vi "Create_Raw_data_file.vi"(4 "No of averages":i32=1, 5 "End time":dbl, 6 "Start time":dbl, 7 "Setup filename":string) -> (0 "Error String":string, 1 "Values":string[][](array[string]), 2 "Header Comments":string[](array[string]), 3 "Column headers":string[](array[string]))   [LabVIEW 2014]
uses:
  File/Setup_Filetype.ctl
  Controls/Post_Process.ctl
  Globals/Preference_global.vi
  Globals/Meas_global.vi
  Globals/Trav_pos_global.vi
  Globals/Constants_global.vi
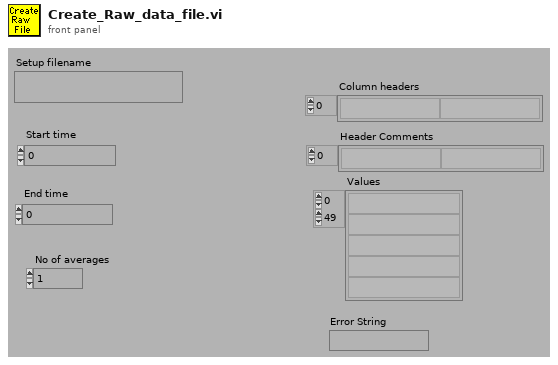
[diagram p1: front panel]
types:
  T1 = typedef "Post_Process.ctl" = enum16{"Take New Data", "Post Process Raw Data File"}
  T2 = typedef "Server_Comms.ctl" = enum16{"Server Link Healthy", "Do Not Link To Server"}
  T3 = typedef "Setup_Filetype.ctl" = enum16{"Measurement Setups", "Calibration Setups", "General", "Results File Plotter Setups", "Speed Calib Tweaks"}
  T4 = typedef "Traverse_cluster.ctl" = cluster{"Start X":sgl, "Start Y":sgl, "Start Z":sgl, "End X":sgl, "End Y":sgl, "End Z":sgl, "No. of pts.":i32, "Spacing":T5, "Filename":path, "Tunnel Speed":dbl, "Averaging time (min)":dbl, "Extra Commands":string, "Carrier_1 Q (l/min)":dbl, "Carrier_2 Q (l/min)":dbl, "Trace Gas Concentration (%)":dbl, "Specific Arguments":string, "Comments":string, "Row No":i32, "Row Type Selector":T6, "Completion time":string, "Row Duration (mins)":dbl, "No. of Valid pts.":i32, "Meas Setup File":string}
  T5 = typedef "Spacing.ctl" = enum16{"Linear", "Log", "Gauss", "Specified", "N/A"}
  T6 = typedef "Multi_run_mode.ctl" = enum16{"Move Traverse Only", "Set Tunnel Speed Only", "Set Source Only", "Set Measurement Conditions", "Single Measurement", "Vertical Profile", "Lateral Profile", "Longitudinal Profile", "Explore Volume", "Multi-Axis Profile", "Auto Calibrate", "Meas Fast FID Bkgnd", "Check Beam Power", "Scanning Valve Measurement", "Run VI Named:", "Set ADAM Ch", "Wait (minutes)", "Send Message", "Synchronize With:", "Fall Back to this Row", "Turn Off Row Repeating", "Blank Row", "Traverse 3D Volume"}
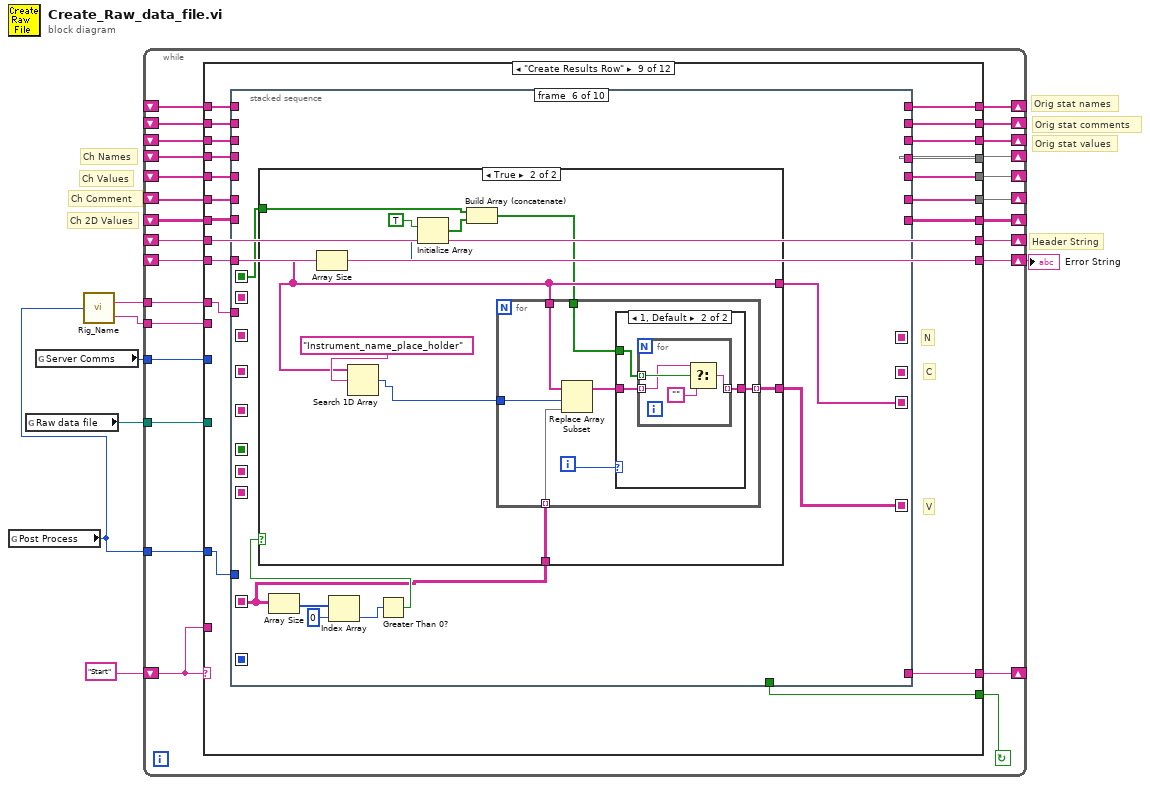
[diagram p0: block diagram]
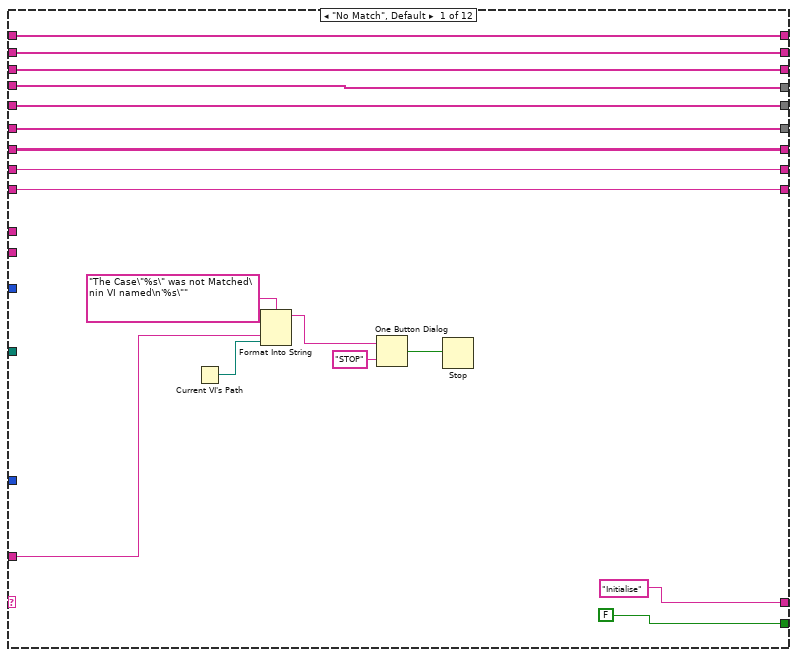
[diagram p2: hidden frame]
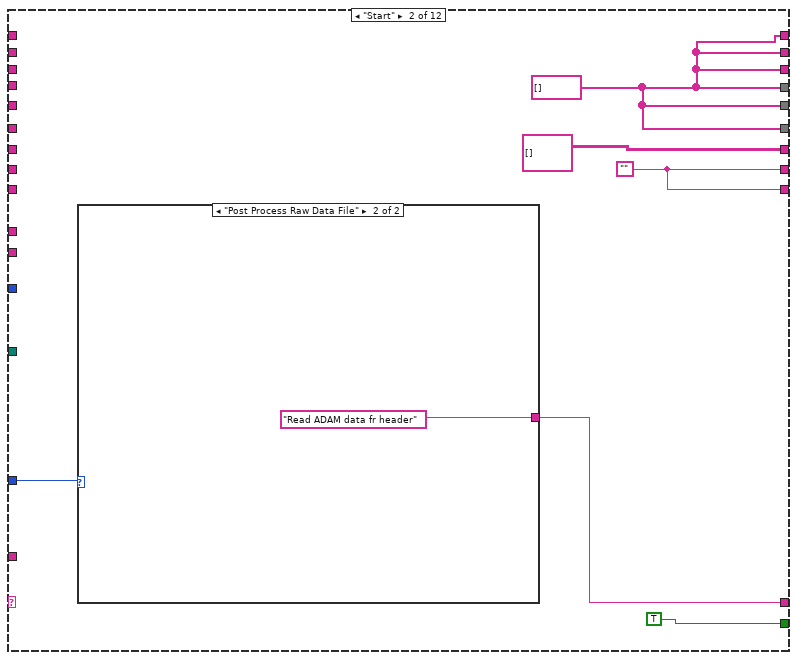
[diagram p3: hidden frame]
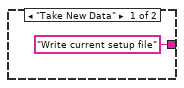
[diagram p4: hidden frame]
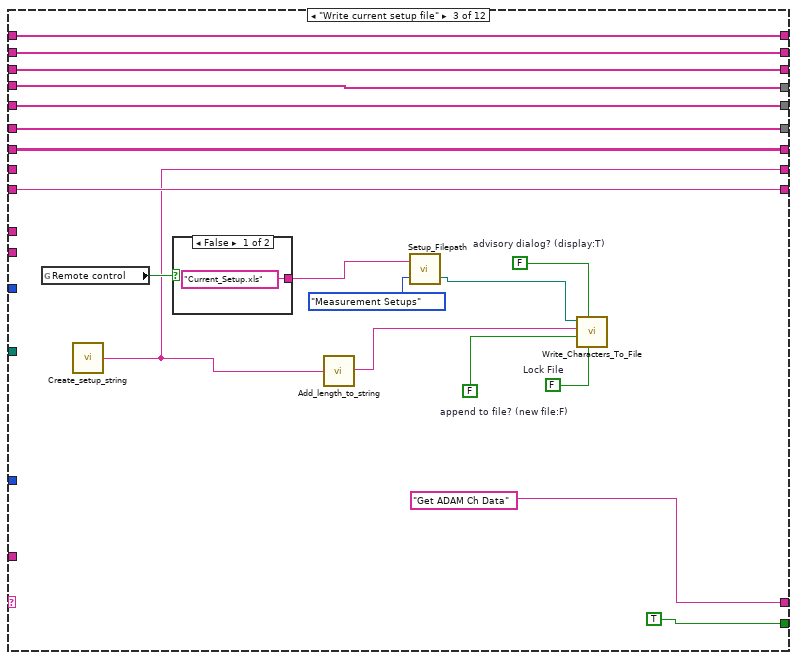
[diagram p5: hidden frame]
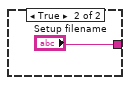
[diagram p6: hidden frame]
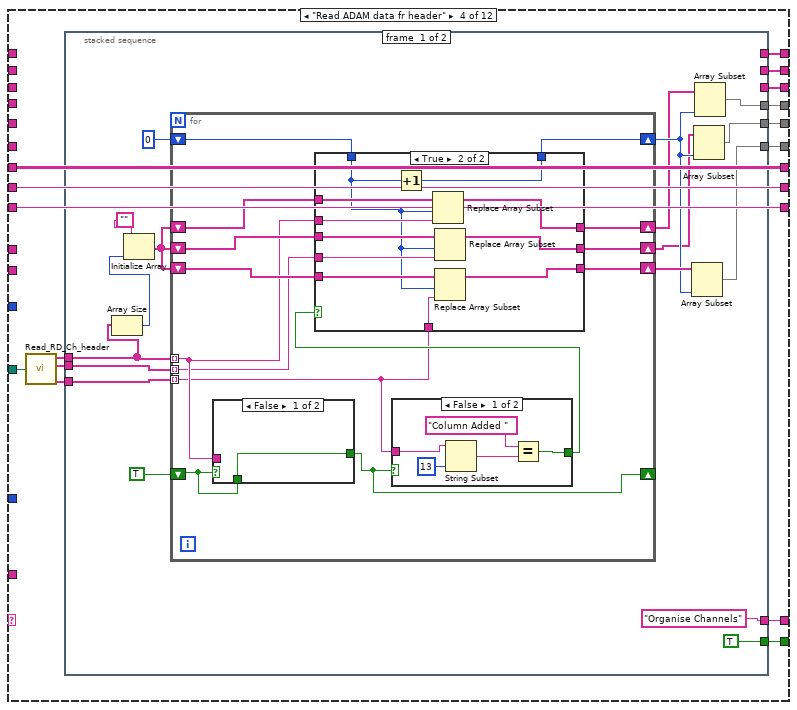
[diagram p7: hidden frame]
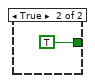
[diagram p9: hidden frame]
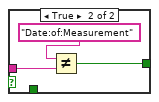
[diagram p10: hidden frame]
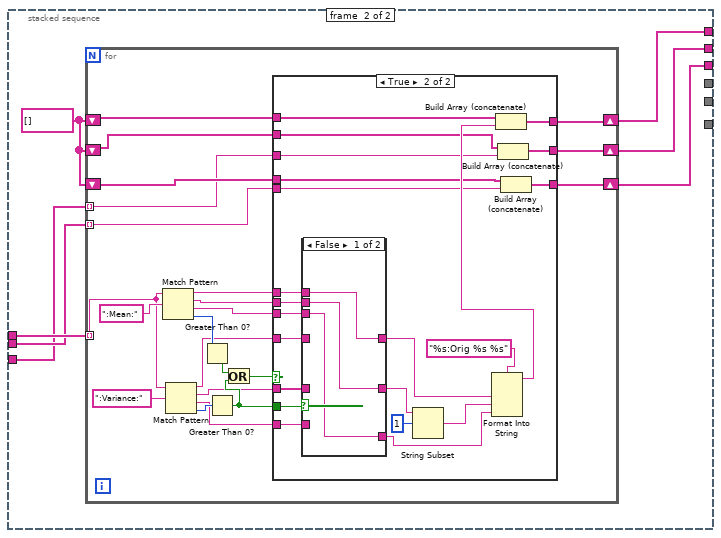
[diagram p11: hidden frame]
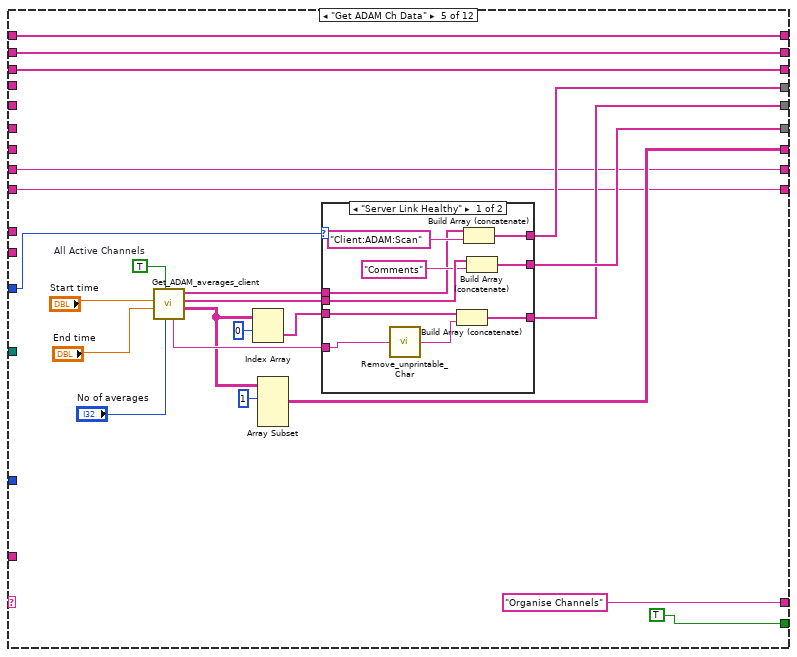
[diagram p14: hidden frame]
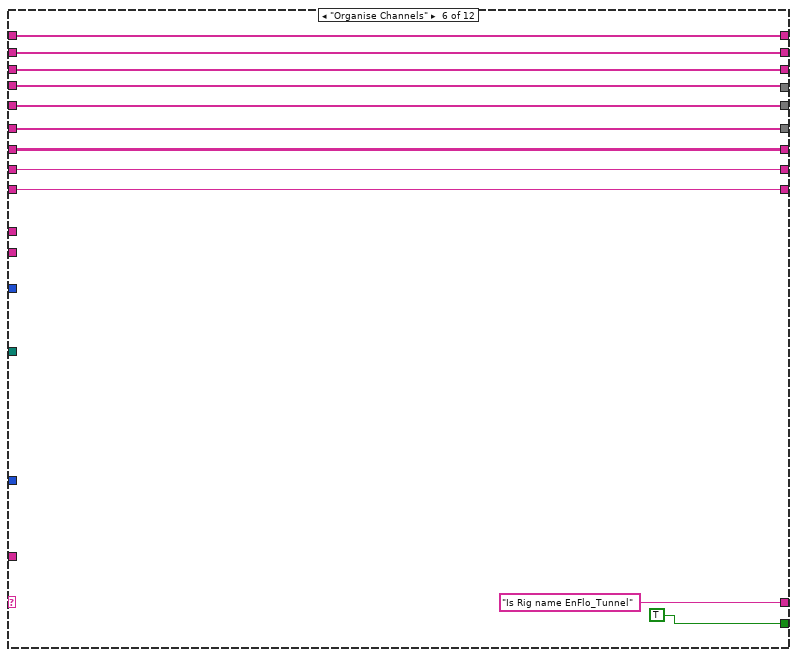
[diagram p16: hidden frame]
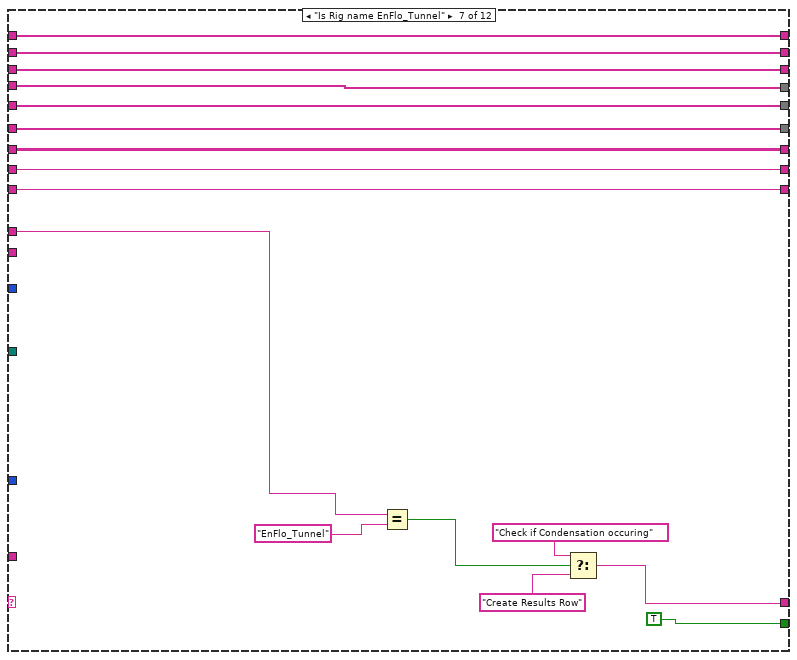
[diagram p17: hidden frame]
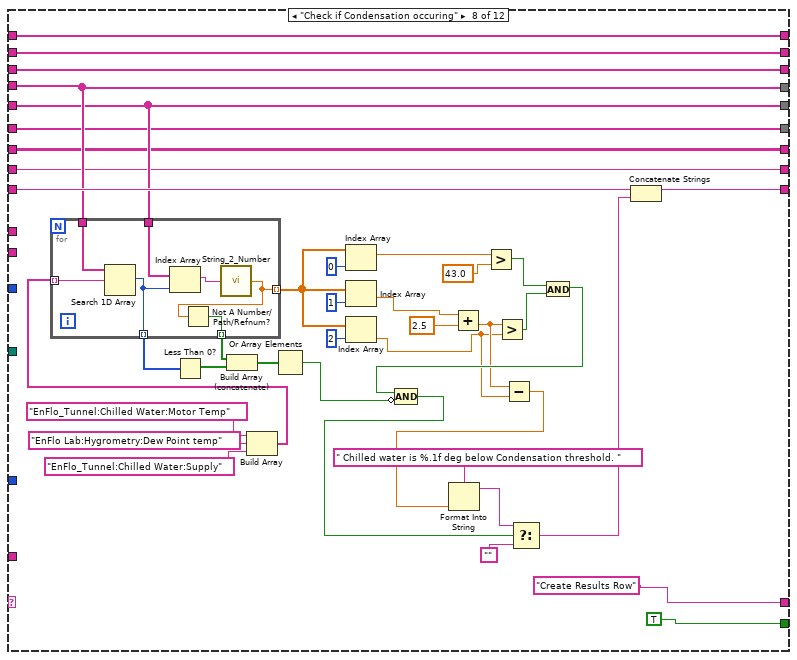
[diagram p18: hidden frame]
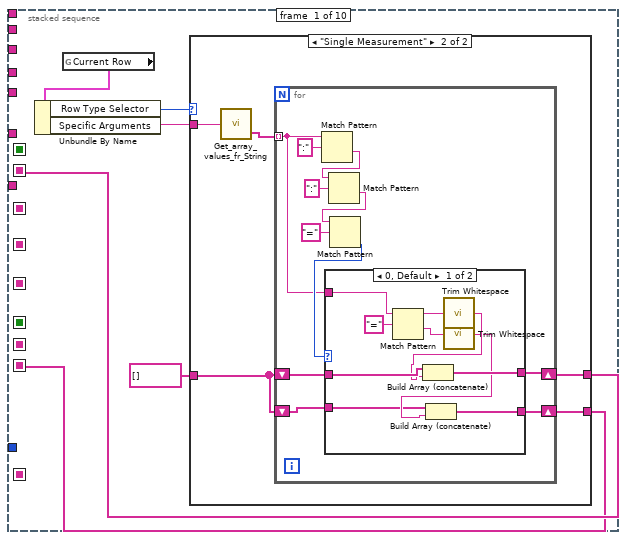
[diagram p19: hidden frame]
diagram:
  # "Orig stat values"
  # "Orig stat comments"
  # "Orig stat names"
  # "Header String"
  # "Ch 2D Values"
  # "Ch Comment"
  # "Ch Values"
  # "Ch Names"
  n1 = global read "Meas_global.vi" "Post Process"() -> (w3:T1)
  n2 = global read "Meas_global.vi" "Raw data file"() -> (w6:path)
  n3 = global read "Preference_global.vi" "Server Comms"() -> (w5:T2)
  n4 = call "Rig_Name.vi"("Post Process"=w3) -> ("Rig Setup before dash"=w2:string, "Hard Disk name"=w1:string)
  n5 = while {
    tunnel: w5 -> [w16]
    tunnel: w6 -> [w17]
    tunnel: w3 -> [w18]
    shift-left: _ -> [w20]
    shift-right: [w19] -> _
    shift-left: _ -> [w26]
    shift-right: [w25] -> w4
    shift-left: _ -> [w21]
    shift-right: [w27] -> _
    shift-left: _ -> [w22]
    shift-right: [w29] -> _
    shift-left: _ -> [w23]
    shift-right: [w28] -> _
    shift-left: _ -> [w24]
    shift-right: [w30] -> _
    shift-left: "Start" -> [w31]
    shift-right: [w32] -> _
    tunnel: w2 -> [w15]
    tunnel: w1 -> [w14]
    shift-right: [w10] -> _
    shift-left: _ -> [w11]
    shift-right: [w8] -> _
    shift-left: _ -> [w9]
    shift-right: [w12] -> _
    shift-left: _ -> [w13]
    stop <- w33 continue-if-true
    n6 = case shown="\"Create Results Row\"" w31 {
      tunnel: [FALSE TRUE TRUE w83 TRUE TRUE TRUE TRUE w328 TRUE TRUE FALSE] -> w33
      tunnel: ["Initialise" w52 "Get ADAM Ch Data" w94 "Organise Channels" "Is Rig name EnFlo_Tunnel" w265 "Create Results Row" w340 "Add Raw Data header info" "Add Raw Data fr Tempory file" "End"] -> w32
      tunnel: w31 -> [w45 _ _ _ _ _ _ _ _ _ _ _]
      tunnel: [w42 w51 w77 w85 w221 w255 w273 w283 w337 w643 w673 w690] -> w30
      tunnel: [w40 w51 w75 w86 w220 w253 w271 w281 w334 w654 w675 w692] -> w29
      tunnel: [w41 w51 w76 w84 w219 w254 w272 w282 w330 w655 w674 w691] -> w28
      tunnel: [w39 string[][] [] w74 w92 w217 w252 w270 w280 w332 w646 w676 w693] -> w27
      tunnel: w26 -> [w38 _ w72 w93 w216 w250 w267 w286 w338 w659 w677 w694]
      tunnel: [w38 w54 w72 w93 w216 w250 w267 w284 w338 w659 w677 w694] -> w25
      tunnel: w24 -> [w42 _ w77 _ _ w255 w273 w283 w336 w643 w673 w690]
      tunnel: w23 -> [w41 _ w76 _ _ w254 w272 w282 w331 w655 w674 w691]
      tunnel: w22 -> [w40 _ w75 _ _ w253 w271 w281 w335 w654 w675 w692]
      tunnel: w21 -> [w39 _ w74 w92 _ w252 w270 w280 w333 w646 w676 w693]
      tunnel: w20 -> [w37 _ _ w91 w215 w251 w268 w278 w339 w648 w670 w689]
      tunnel: [w37 w54 w66 w91 w215 w251 w268 w278 w339 w651 w669 ""] -> w19
      tunnel: w18 -> [_ w53 _ _ _ _ _ _ w329 _ _ _]
      tunnel: w17 -> [_ _ _ w90 _ _ _ _ _ _ _ w685]
      tunnel: w16 -> [_ _ _ _ w214 _ _ _ _ _ _ _]
      tunnel: w15 -> [_ _ _ _ _ _ w262 _ w327 _ _ _]
      tunnel: w14 -> [_ _ _ _ _ _ _ _ _ _ _ _]
      tunnel: w13 -> [w36 _ w64 _ w213 w249 w260 w277 w325 w640 w668 w682]
      tunnel: [w36 w51 w64 w82 w213 w249 w260 w277 w326 w640 w668 w682] -> w12
      tunnel: w11 -> [w35 _ w63 _ w212 w248 w259 w276 w324 w639 w667 w681]
      tunnel: [w35 w51 w63 w81 w212 w248 w259 w276 w323 w639 w667 w681] -> w10
      tunnel: w9 -> [w34 _ w62 _ w211 w247 w258 w275 w321 w638 w666 w680]
      tunnel: [w34 w51 w62 w80 w211 w247 w258 w275 w322 w638 w666 w680] -> w8
      frame "No Match", Default {
        n7 = Current VI's Path() -> (path=w44:path)
        n8 = Format Into String(format string="The Case\"%s\" was not Matched\nin VI named\n'%s\"" ("Format String"), w45, w44) -> (resulting string=w48:string)  [unwired: 2 in, 1 out]
        n9 = One Button Dialog(message=w48, button name ("OK")="STOP") -> (true=w46:bool)
        n10 = Stop(stop? (T)=w46) -> ()
      }
      frame "Start" {
        w54 = ""
        w51 = string[] []
        n11 = case shown="\"Post Process Raw Data File\"" w53 {
          tunnel: ["Write current setup file" "Read ADAM data fr header"] -> w52
          frame "Take New Data" {
          }
          frame "Post Process Raw Data File" {
          }
        }
      }
      frame "Write current setup file" {
        w67 = FALSE  # Lock File
        w70 = FALSE  # advisory dialog? (display:T)
        w71 = FALSE  # append to file? (new file:F)
        n12 = global read "Meas_global.vi" "Remote control"() -> (w69:bool)
        n13 = call "Create_setup_string.vi"() -> ("Setup String"=w66:string)  [unwired: 1 out]
        n14 = case shown="False" w69 {
          tunnel: ["Current_Setup.xls" ("Setup filename") "Setup filename"] -> w60
          frame False {
          }
          frame True {
          }
        }
        n15 = call "Add_length_to_string.vi"("String in"=w66) -> ("String out"=w68:string)
        n16 = call "Setup_Filepath.vi"("Setup File Type"=Setup_Filetype."Measurement Setups", "Filename in"=w60) -> ("Filename Out"=w59:path)  [unwired: 1 out]
        n17 = call "Write_Characters_To_File.vi"("file path (dialog if empty)"=w59, "advisory dialog? (display:T)"=w70, "character string"=w68, "append to file? (new file:F)"=w71, "Lock File"=w67) -> ()  [unwired: 4 out]
      }
      frame "Read ADAM data fr header" {
        n18 = call "Read_RD_Ch_header.vi"("Raw data file"=w90) -> ("Ch Name Out"=w88:string[], "Ch Values"=w87:string[], "Comments"=w89:string[])  [unwired: 1 out]
        n19 = stacked-sequence {
          tunnel: ["Organise Channels" _] -> w94
          tunnel: w89 -> [w109 w154]
          tunnel: w88 -> [w108 w157]
          tunnel: w87 -> [w103 w155]
          tunnel: [w100 _] -> w86
          tunnel: [w97 _] -> w85
          tunnel: [w96 _] -> w84
          tunnel: [TRUE _] -> w83
          tunnel: [_ w153] -> w82
          tunnel: [_ w152] -> w81
          tunnel: [_ w151] -> w80
          frame #0 {
            n20 = Array Size(array=w108) -> (size(s)=w106:i32)
            n21 = Initialize Array("", w106) -> (w105:string[])
            n22 = for {
              shift-right: [w112] -> w101
              shift-left: 0 -> [w122]
              shift-right: [w116] -> w102
              shift-left: w105 -> [w119]
              shift-right: [w117] -> w99
              shift-left: w105 -> [w120]
              shift-right: [w118] -> w98
              shift-left: w105 -> [w121]
              shift-right: [w124] -> _
              shift-left: TRUE -> [w125]
              tunnel: w108 -> [w115] mode=indexing
              tunnel: w109 -> [w113] mode=indexing
              tunnel: w103 -> [w114] mode=indexing
              n23 = case shown="False" w125 {
                tunnel: w115 -> [_ w150]
                tunnel: [w147 w148] -> w124
                tunnel: w125 -> [w147 _]
                frame False {
                }
                frame True {
                  n24 = Not Equal?(x="Date:of:Measurement", y=w150) -> (x != y?=w148:bool)
                }
              }
              n25 = case shown="False" w124 {
                tunnel: w113 -> [w142 _]
                tunnel: [w144 TRUE] -> w123
                frame False {
                  n26 = String Subset(string=w142, length (rest)=13 ("length (rest)")) -> (substring=w141:string)  [unwired: 1 out]
                  n27 = Equal?(x="Column Added ", y=w141) -> (x = y?=w144:bool)
                }
                frame True {
                }
              }
              n28 = case shown="True" w123 {
                tunnel: w122 -> [w126 w131]
                tunnel: w121 -> [w129 w140]
                tunnel: w120 -> [w128 w139]
                tunnel: w119 -> [w127 w138]
                tunnel: [w129 w137] -> w118
                tunnel: [w128 w136] -> w117
                tunnel: [w127 w135] -> w116
                tunnel: w115 -> [_ w134]
                tunnel: w114 -> [_ w133]
                tunnel: w113 -> [_ w132]
                tunnel: [w126 w130] -> w112
                frame False {
                }
                frame True {
                  n29 = Increment(x=w131) -> (x+1=w130:i32)
                  n30 = Replace Array Subset(array=w140, new element=w134, index=w131) -> (w137:string[])
                  n31 = Replace Array Subset(array=w139, new element=w133, index=w131) -> (w136:string[])
                  n32 = Replace Array Subset(array=w138, new element=w132, index=w131) -> (w135:string[])
                }
              }
            }
            n33 = Array Subset(array=w102, length=w101) -> (w100:string[])  [unwired: 1 in]
            n34 = Array Subset(array=w99, length=w101) -> (w96:string[])  [unwired: 1 in]
            n35 = Array Subset(array=w98, length=w101) -> (w97:string[])  [unwired: 1 in]
          }
          frame #1 {
            w156 = string[] []
            n36 = for {
              shift-right: [w165] -> w153
              shift-left: w156 -> [w164]
              shift-right: [w158] -> w152
              shift-left: w156 -> [w159]
              shift-right: [w161] -> w151
              shift-left: w156 -> [w162]
              tunnel: w157 -> [w177] mode=indexing
              tunnel: w155 -> [w163] mode=indexing
              tunnel: w154 -> [w160] mode=indexing
              n37 = Match Pattern(string=w177, regular expression=":Mean:") -> (before substring=w168:string, match substring=w167:string, after substring=w166:string, offset past match=w176:i32)  [unwired: 1 out]
              n38 = Match Pattern(string=w177, regular expression=":Variance:") -> (before substring=w171:string, match substring=w170:string, after substring=w169:string, offset past match=w175:i32)  [unwired: 1 out]
              n39 = Greater Than 0?(x=w176) -> (x > 0?=w174:bool)
              n40 = Greater Than 0?(x=w175) -> (x > 0?=w172:bool)
              n41 = Or(x=w174, y=w172) -> (x .or. y?=w173:bool)
              n42 = case shown="True" w173 {
                tunnel: w172 -> [_ w204]
                tunnel: w171 -> [_ w203]
                tunnel: w170 -> [_ w202]
                tunnel: w169 -> [_ w201]
                tunnel: w168 -> [_ w194]
                tunnel: w167 -> [_ w193]
                tunnel: w166 -> [_ w192]
                tunnel: [w182 w190] -> w165
                tunnel: w164 -> [w182 w189]
                tunnel: w163 -> [_ w188]
                tunnel: w162 -> [w180 w187]
                tunnel: [w180 w186] -> w161
                tunnel: w160 -> [_ w185]
                tunnel: w159 -> [w181 w184]
                tunnel: [w181 w183] -> w158
                frame False {
                }
                frame True {
                  n43 = case shown="False" w204 {
                    tunnel: w203 -> [_ w209]
                    tunnel: w202 -> [_ w210]
                    tunnel: w201 -> [_ w208]
                    tunnel: [w206 w210] -> w199
                    tunnel: [w207 w209] -> w196
                    tunnel: [w205 w208] -> w195
                    tunnel: w194 -> [w207 _]
                    tunnel: w193 -> [w206 _]
                    tunnel: w192 -> [w205 _]
                    frame False {
                    }
                    frame True {
                    }
                  }
                  n44 = String Subset(string=w199, offset (0)=1) -> (substring=w198:string)  [unwired: 1 out]
                  n45 = Format Into String(format string="%s:Orig %s %s", w196, w198, w195) -> (resulting string=w191:string)  [unwired: 2 in, 1 out]
                  n46 = Build Array (concatenate)(w189, w191) -> (w190:string[])
                  n47 = Build Array (concatenate)(w184, w185) -> (w183:string[])
                  n48 = Build Array (concatenate)(w187, w188) -> (w186:string[])
                }
              }
            }
          }
        }
      }
      frame "Get ADAM Ch Data" {
        w224 = TRUE  # All Active Channels
        n49 = call "Get_ADAM_averages_client.vi"("No of averages"="No of averages", "All Active Channels"=w224, "End time"="End time", "Start time"="Start time") -> ("Values"=w227:string[][], "Comments"=w230:string[], "Titles"=w229:string[], "Messages"=w231:string)  [unwired: 1 in, 3 out]
        n50 = Index Array(array=w227, index (row)=0 ("Index")) -> (element=w218:string[])  [unwired: 1 in]
        n51 = Array Subset(array=w227, index (row)=1 ("Array Index")) -> (w217:string[][])  [unwired: 3 in]
        n52 = case shown="\"Server Link Healthy\"" w214 {
          tunnel: w231 -> [w235 _]
          tunnel: w230 -> [w243 w245]
          tunnel: w229 -> [w240 w246]
          tunnel: [w239 w246] -> w221
          tunnel: [w238 w245] -> w220
          tunnel: [w237 w244] -> w219
          tunnel: w218 -> [w236 w244]
          frame "Server Link Healthy" {
            n53 = call "Remove_unprintable_Char.vi"("Input String"=w235) -> ("Output String"=w234:string)
            n54 = Build Array (concatenate)(w236, w234) -> (w237:string[])
            n55 = Build Array (concatenate)(w240, "Client:ADAM:Scan") -> (w239:string[])
            n56 = Build Array (concatenate)(w243, "Comments" ("Comments")) -> (w238:string[])
          }
          frame "Do Not Link To Server" {
          }
        }
      }
      frame "Organise Channels" {
      }
      frame "Is Rig name EnFlo_Tunnel" {
        n57 = Equal?(x=w262, y="EnFlo_Tunnel") -> (x = y?=w266:bool)
        n58 = Select(t="Check if Condensation occuring", s=w266, f="Create Results Row") -> (s? t:f=w265:string)
      }
      frame "Check if Condensation occuring" {
        n59 = Build Array("EnFlo_Tunnel:Chilled Water:Motor Temp", "EnFlo Lab:Hygrometry:Dew Point temp", "EnFlo_Tunnel:Chilled Water:Supply") -> (w309:string[])
        n60 = for {
          tunnel: w283 -> [w320]
          tunnel: w309 -> [w319] mode=indexing
          tunnel: w282 -> [w318]
          tunnel: [w316] -> w310 mode=indexing
          tunnel: [w315] -> w308 mode=indexing
          tunnel: [w314] -> w301 mode=indexing
          n61 = Search 1D Array(1D array=w320, element=w319) -> (index of element=w316:i32)  [unwired: 1 out]
          n62 = Index Array(array=w318, index=w316) -> (element=w317:string)
          n63 = call "String_2_Number.vi"("Value"=w317) -> ("Numeric"=w315:dbl)
          n64 = Not A Number/Path/Refnum?(number/path/refnum=w315) -> (NaN/Path/Refnum?=w314:bool)
        }
        n65 = Less Than 0?(x=w310) -> (x < 0?=w300:bool[])
        n66 = Build Array (concatenate)(w301, w300) -> (w299:bool[])
        n67 = Or Array Elements(Boolean array=w299) -> (logical OR=w295:bool)
        n68 = Index Array(array=w308, index=0 ("Index")) -> (element=w302:dbl)
        n69 = Index Array(array=w308, index=1 ("Index")) -> (element=w298:dbl)
        n70 = Index Array(array=w308, index=2 ("Index")) -> (element=w290:dbl)
        n71 = Add(x=w298, y=2.5) -> (x+y=w291:dbl)
        n72 = Greater?(x=w302, y=43.0) -> (0:w296:bool)
        n73 = Greater?(x=w291, y=w290) -> (0:w297:bool)
        n74 = Subtract(x=w291, y=w290) -> (x-y=w289:dbl)
        n75 = Format Into String(format string=" Chilled water is %.1f deg below Condensation threshold. " ("Format String"), w289) -> (resulting string=w287:string)  [unwired: 2 in, 1 out]
        n76 = And(x=w296, y=w297) -> (x .and. y?=w294:bool)
        n77 = Compound Arithmetic op=AND(w294, invert w295) -> (w293:bool)
        n78 = Select(t=w287, s=w293, f="") -> (s? t:f=w285:string)
        n79 = Concatenate Strings(w286, w285) -> (w284:string)
      }
      frame "Create Results Row" {
        # "V"
        # "C"
        # "N"
        n80 = stacked-sequence {
          seq-local: [_ w379 _ _ _ _ _ _ _ _] -> [_ _ _ w421 w462 _ _ _ _ _]
          seq-local: [_ w378 _ _ _ _ _ _ _ _] -> [_ _ _ w417 w461 _ _ _ _ _]
          seq-local: [_ _ w401 _ _ _ _ _ _ _] -> [_ _ _ w415 w460 _ _ _ _ _]
          seq-local: [_ w386 _ _ _ _ _ _ _ _] -> [_ _ _ _ _ w498 _ _ _ _]
          seq-local: [_ _ _ _ w459 _ _ _ _ _] -> [_ _ _ _ _ w500 _ _ _ _]
          seq-local: [w342 _ _ _ _ _ _ _ _ _] -> [_ w382 _ _ _ _ _ _ _ _]
          seq-local: [w341 _ _ _ _ _ _ _ _ _] -> [_ _ w403 _ _ _ _ _ _ _]
          seq-local: [_ _ _ _ w458 _ _ _ _ _] -> [_ _ _ _ _ _ _ w571 w609 _]
          seq-local: [_ _ _ _ w457 _ _ _ _ _] -> [_ _ _ _ _ _ _ _ w607 _]
          seq-local: [_ _ _ _ _ w497 _ _ _ _] -> [_ _ _ _ _ _ _ _ w606 _]
          seq-local: [_ _ _ _ _ _ w531 _ _ _] -> [_ _ _ _ _ _ _ w570 w610 _]
          seq-local: [_ _ _ _ _ _ _ w569 _ _] -> [_ _ _ _ _ _ _ _ w608 _]
          seq-local: [_ w377 _ _ _ _ _ _ _ _] -> [_ _ w402 _ _ _ _ _ _ _]
          seq-local: [_ w376 _ _ _ _ _ _ _ _] -> [_ _ _ _ _ w496 _ _ _ _]
          tunnel: [_ _ "Add Adam Chs to header" _ _ _ _ _ _ _] -> w340
          tunnel: w336 -> [_ w385 _ w419 _ _ w534 _ _ _]
          tunnel: w335 -> [_ w384 _ w420 _ _ _ _ _ _]
          tunnel: w338 -> [_ _ w406 _ _ _ _ _ _ _]
          tunnel: w331 -> [_ _ w405 w414 _ _ w533 _ _ _]
          tunnel: w333 -> [_ _ w404 _ _ _ _ _ _ _]
          tunnel: [_ _ _ w418 _ _ _ _ _ _] -> w337
          tunnel: [_ _ _ w416 _ _ _ _ _ _] -> w334
          tunnel: [_ _ w404 _ _ _ _ _ _ _] -> w332
          tunnel: [_ _ _ w413 _ _ _ _ _ _] -> w330
          tunnel: w329 -> [_ _ _ w412 w463 _ w541 _ _ _]
          tunnel: [_ _ _ _ _ _ w537 _ _ _] -> w328
          tunnel: w327 -> [_ _ _ _ _ _ w535 _ _ _]
          tunnel: [_ _ _ _ _ _ _ _ _ w637] -> w326
          tunnel: w325 -> [_ _ _ _ _ _ _ _ w604 w637]
          tunnel: w324 -> [_ _ _ _ _ _ _ _ w601 w636]
          tunnel: [_ _ _ _ _ _ _ _ _ w636] -> w323
          tunnel: [_ _ _ _ _ _ _ _ _ w635] -> w322
          tunnel: w321 -> [_ _ _ _ _ _ _ _ w598 w635]
          frame #0 {
            n81 = global read "Trav_pos_global.vi" "Current Row"() -> (w346:T4)
            n82 = Unbundle By Name(w346) -> ("Row Type Selector"=w345:T6, "Specific Arguments"=w344:string)
            n83 = case shown="\"Single Measurement\"" w345 {
              tunnel: w344 -> [_ w352]
              tunnel: string[] [] -> [w347 w350]
              tunnel: [w347 w349] -> w342
              tunnel: [w347 w348] -> w341
              frame "Move Traverse Only", Default {
              }
              frame "Single Measurement" {
                n84 = call "Get_array_values_fr_String.vi"("String Value"=w352) -> ("String array"=w351:string[])  [unwired: 1 out]
                n85 = for {
                  tunnel: w351 -> [w355] mode=indexing
                  shift-right: [w353] -> w348
                  shift-left: w350 -> [w354]
                  shift-right: [w356] -> w349
                  shift-left: w350 -> [w357]
                  n86 = Match Pattern(string=w355, regular expression=":") -> (after substring=w361:string)  [unwired: 4 out]
                  n87 = Match Pattern(string=w361, regular expression=":") -> (after substring=w359:string)  [unwired: 4 out]
                  n88 = Match Pattern(string=w359, regular expression="=") -> (offset past match=w358:i32)  [unwired: 4 out]
                  n89 = case shown="0, Default" w358 {
                    tunnel: w357 -> [w373 w375]
                    tunnel: [w372 w375] -> w356
                    tunnel: w355 -> [w368 _]
                    tunnel: w354 -> [w365 w374]
                    tunnel: [w364 w374] -> w353
                    frame 0, Default {
                      n90 = Match Pattern(string=w368, regular expression="=") -> (before substring=w370:string, after substring=w369:string)  [unwired: 3 out]
                      n91 = call <vilib>:"Trim Whitespace.vi"("string"=w370) -> ("trimmed string"=w367:string)  [unwired: 1 in]
                      n92 = Build Array (concatenate)(w373, w367) -> (w372:string[])
                      n93 = call <vilib>:"Trim Whitespace.vi"("string"=w369) -> ("trimmed string"=w366:string)  [unwired: 1 in]
                      n94 = Build Array (concatenate)(w365, w366) -> (w364:string[])
                    }
                    frame -1 {
                    }
                  }
                }
              }
            }
          }
          frame #1 {
            n95 = for {
              tunnel: w385 -> [w399] mode=indexing
              tunnel: w384 -> [w398] mode=indexing
              tunnel: [w397] -> w381 mode=indexing
              n96 = Concatenate Strings(w399, ":" ("Substring"), w398) -> (w397:string)
            }
            n97 = call "Create_Results_Row.vi"() -> ("row splitting"=w386:string[][], "Values to Keep in Dup rows"=w376:bool[], "Channel Values"=w377:string[], "Channel Names"=w383:string[])  [unwired: 5 in]
            n98 = Build Array (concatenate)(w383, w382, w381) -> (w380:string[])
            n99 = for {
              tunnel: w380 -> [w387] mode=indexing
              tunnel: [w391] -> w379 mode=indexing
              tunnel: [w388] -> w378 mode=indexing
              w390 = ":" ("regular expression")
              n100 = Match Pattern(string=w387, regular expression=w390) -> (before substring=w394:string, after substring=w396:string)  [unwired: 3 out]
              n101 = Match Pattern(string=w396, regular expression=w390) -> (before substring=w393:string, after substring=w395:string)  [unwired: 3 out]
              n102 = Match Pattern(string=w395, regular expression=w390) -> (before substring=w392:string, after substring=w389:string)  [unwired: 3 out]
              n103 = Match Pattern(string=w389, regular expression=w390) -> (before substring=w388:string)  [unwired: 4 out]
              n104 = Concatenate Strings(w394, w390, w393, w390, w392) -> (w391:string)
            }
          }
          frame #2 {
            w407 = 5  # Comment Column
            n105 = Index Array(array=w402, index=w407) -> (element=w409:string)
            n106 = Concatenate Strings(w409, w406) -> (w410:string)
            n107 = Replace Array Subset(array=w402, new element=w410, index=w407) -> (w408:string[])
            n108 = Build Array (concatenate)(w408, w403, w405) -> (w401:string[])
          }
          frame #3 {
            n109 = case shown="\"Take New Data\"" w412 {
              tunnel: w421 -> [w430 _]
              tunnel: w420 -> [w429 w455]
              tunnel: w419 -> [w428 w456]
              tunnel: [w427 w456] -> w418
              tunnel: w417 -> [w426 _]
              tunnel: [w425 w455] -> w416
              tunnel: w415 -> [w424 _]
              tunnel: w414 -> [w423 w454]
              tunnel: [w422 w454] -> w413
              frame "Take New Data" {
                n110 = for {
                  tunnel: w428 -> [w441]
                  tunnel: w430 -> [w437] mode=indexing
                  shift-right: [w438] -> w427
                  shift-left: w428 -> [w439]
                  shift-right: [w435] -> w425
                  shift-left: w429 -> [w436]
                  shift-right: [w432] -> w422
                  shift-left: w423 -> [w433]
                  tunnel: w426 -> [w434] mode=indexing
                  tunnel: w424 -> [w431] mode=indexing
                  n111 = Search 1D Array(1D array=w441, element=w437) -> (index of element=w440:i32)  [unwired: 1 out]
                  n112 = case shown="-1" w440 {
                    tunnel: w439 -> [w444 w453]
                    tunnel: [w444 w451] -> w438
                    tunnel: w437 -> [_ w452]
                    tunnel: w436 -> [w443 w450]
                    tunnel: [w443 w449] -> w435
                    tunnel: w434 -> [_ w448]
                    tunnel: w433 -> [w442 w446]
                    tunnel: [w442 w445] -> w432
                    tunnel: w431 -> [_ w447]
                    frame 0, Default {
                    }
                    frame -1 {
                      n113 = Build Array (concatenate)(w446, w447) -> (w445:string[])
                      n114 = Build Array (concatenate)(w453, w452) -> (w451:string[])
                      n115 = Build Array (concatenate)(w450, w448) -> (w449:string[])
                    }
                  }
                }
              }
              frame "Post Process Raw Data File" {
              }
            }
          }
          frame #4 {
            # "Values"
            # "Comments"
            # "Ch Names"
            n116 = case shown="\"Post Process Raw Data File\"" w463 {
              tunnel: [w466 w472] -> w458
              tunnel: w462 -> [w466 w473]
              tunnel: [w465 w471] -> w457
              tunnel: w461 -> [w465 w469]
              tunnel: [w464 w470] -> w459
              tunnel: w460 -> [w464 w468]
              frame "Take New Data" {
              }
              frame "Post Process Raw Data File" {
                w467 = string[] []
                n117 = for {
                  shift-right: [w481] -> w472
                  shift-left: w467 -> [w482]
                  shift-right: [w476] -> w471
                  shift-left: w467 -> [w479]
                  shift-right: [w477] -> w470
                  shift-left: w467 -> [w478]
                  tunnel: w473 -> [w480] mode=indexing
                  tunnel: w469 -> [w475] mode=indexing
                  tunnel: w468 -> [w474] mode=indexing
                  n118 = Search 1D Array(1D array=w482, element=w480) -> (index of element=w483:i32)  [unwired: 1 out]
                  n119 = case shown="-1" w483 {
                    tunnel: w482 -> [w486 w495]
                    tunnel: [w486 w494] -> w481
                    tunnel: w480 -> [_ w493]
                    tunnel: w479 -> [w485 w492]
                    tunnel: w478 -> [w484 w491]
                    tunnel: [w484 w490] -> w477
                    tunnel: [w485 w489] -> w476
                    tunnel: w475 -> [_ w488]
                    tunnel: w474 -> [_ w487]
                    frame 0, Default {
                    }
                    frame -1 {
                      n120 = Build Array (concatenate)(w495, w493) -> (w494:string[])
                      n121 = Build Array (concatenate)(w492, w488) -> (w489:string[])
                      n122 = Build Array (concatenate)(w491, w487) -> (w490:string[])
                    }
                  }
                }
              }
            }
          }
          frame #5 {
            n123 = Array Size(array=w498) -> (size(s)=w503:i32[])
            n124 = Index Array(array=w503, index=0) -> (element=w501:i32)
            n125 = Greater Than 0?(x=w501) -> (x > 0?=w499:bool)
            n126 = case shown="True" w499 {
              tunnel: w500 -> [w505 w511]
              tunnel: w498 -> [_ w513]
              tunnel: [w504 w512] -> w497
              tunnel: w496 -> [_ w507]
              frame False {
                n127 = Build Array(w505) -> (w504:string[][])
              }
              frame True {
                n128 = Array Size(array=w511) -> (size(s)=w510:i32)
                n129 = Search 1D Array(1D array=w511, element="Instrument_name_place_holder") -> (index of element=w514:i32)  [unwired: 1 out]
                n130 = Initialize Array(TRUE, w510) -> (w508:bool[])
                n131 = Build Array (concatenate)(w507, w508) -> (w506:bool[])
                n132 = for {
                  tunnel: w511 -> [w522]
                  tunnel: w514 -> [w521]
                  tunnel: w513 -> [w520] mode=indexing
                  tunnel: [w517] -> w512 mode=indexing
                  tunnel: w506 -> [w516]
                  i -> [w519]
                  n133 = Replace Array Subset(array=w522, new element=w520, index=w521) -> (w518:string[])
                  n134 = case shown="1, Default" w519 {
                    tunnel: w518 -> [w523 w525]
                    tunnel: [w523 w524] -> w517
                    tunnel: w516 -> [_ w526]
                    frame 0 {
                    }
                    frame 1, Default {
                      n135 = for {
                        tunnel: w526 -> [w530] mode=indexing
                        tunnel: w525 -> [w529] mode=indexing
                        tunnel: [w528] -> w524 mode=indexing
                        n136 = Select(t=w529, s=w530, f="") -> (s? t:f=w528:string)
                      }
                    }
                  }
                }
              }
            }
          }
          frame #6 {
            n137 = Equal?(x="EnFlo_Tunnel", y=w535) -> (x = y?=w532:bool)
            n138 = case shown="True" w532 {
              tunnel: w534 -> [_ w550]
              tunnel: w533 -> [_ w547]
              tunnel: [FALSE w545] -> w531
              frame False {
              }
              frame True {
                n139 = disable-structure shown="Enabled" {
                  disable-tunnel: [w551 FALSE] -> w543
                  frame Disabled {
                    n140 = global read "Meas_global.vi" "Pre Setup String"() -> (w555:string)
                    n141 = call "Get_Characters_from_string.vi"("Input string"=w555, "Variable name"="Show_all_EnFlo_Tunnel_Columns") -> ("Status"=w553:enum16{"Char in string", "Char not in string"}, "Value"=w552:string)  [unwired: 1 in]
                    n142 = case shown="\"Char in string\"" w553 {
                      tunnel: w552 -> [w558 _]
                      tunnel: [w556 TRUE] -> w551
                      frame "Char in string" {
                        n143 = Equal?(x=w558, y="TRUE") -> (x = y?=w557:bool)
                        n144 = Not(x=w557) -> (.not. x?=w556:bool)
                      }
                      frame "Char not in string" {
                      }
                    }
                  }
                  frame Enabled {
                  }
                }
                n145 = Search 1D Array(1D array=w550, element="EnFlo_Tunnel:Heater:Enable") -> (index of element=w548:i32)  [unwired: 1 out]
                n146 = case shown="-1" w548 {
                  tunnel: w548 -> [w567 _]
                  tunnel: w547 -> [w566 _]
                  tunnel: [w562 FALSE] -> w546
                  frame 0, Default {
                    n147 = Index Array(array=w566, index=w567) -> (element=w565:string)
                    n148 = call "String_2_Number.vi"("Value"=w565) -> ("Numeric"=w564:dbl)
                    n149 = Less?(x=w564, y=0.5) -> (x < y?=w562:bool)
                  }
                  frame -1 {
                  }
                }
                n150 = Select(t=w546, s=w543, f=FALSE) -> (s? t:f=w545:bool)
              }
            }
            n151 = global read "Trav_pos_global.vi" "Dummy Measurement?"() -> (w538:bool)
            n152 = Equal?(x=Post_Process."Take New Data" ("Post Process"), y=w541) -> (x = y?=w539:bool)
            n153 = Compound Arithmetic op=AND(invert w538, w539) -> (w537:bool)
          }
          frame #7 {
            n154 = case shown="True" w570 {
              tunnel: w571 -> [_ w577]
              tunnel: [i32[] [] w575] -> w569
              frame False {
              }
              frame True {
                w573 = string[] ["EnFlo_Tunnel:Inlet Heater:Temp", "EnFlo_Tunnel:Inlet Rake:Temp", "EnFlo_Tunnel:Trav Thermo:", "EnFlo_Tunnel:floor ", "EnFlo_Tunnel:roof ", "EnFlo_Tunnel:Side ", "EnFlo_Tunnel:Temp:Inlet", "EnFlo_Tunnel:Temp:Floor"] ("Column headers")
                # "Remove these\nChannels"
                # "Remaining\nChannels"
                n155 = for {
                  tunnel: w573 -> [w579] mode=indexing
                  tunnel: [w578] -> w574 mode=indexing
                  n156 = String Length(string=w579) -> (length=w578:i32)
                }
                n157 = for {
                  tunnel: w577 -> [w583] mode=indexing
                  shift-right: [w586] -> w575
                  shift-left: i32[] [] -> [w587]
                  tunnel: w574 -> [w584]
                  tunnel: w573 -> [w582]
                  i -> [w585]
                  n158 = for {
                    tunnel: w584 -> [w592] mode=indexing
                    tunnel: w583 -> [w591]
                    tunnel: w582 -> [w589] mode=indexing
                    tunnel: [w588] -> w581 mode=indexing
                    n159 = String Subset(string=w591, length (rest)=w592) -> (substring=w590:string)  [unwired: 1 out]
                    n160 = Equal?(x=w590, y=w589) -> (x = y?=w588:bool)
                  }
                  n161 = Or Array Elements(Boolean array=w581) -> (logical OR=w580:bool)
                  n162 = case shown="True" w580 {
                    tunnel: w587 -> [w595 w596]
                    tunnel: w585 -> [w594 _]
                    tunnel: [w593 w596] -> w586
                    frame False {
                      n163 = Build Array (concatenate)(w595, w594) -> (w593:i32[])
                    }
                    frame True {
                    }
                  }
                }
              }
            }
          }
          frame #8 {
            n164 = case shown="True" w610 {
              tunnel: w609 -> [w616 w623]
              tunnel: w608 -> [_ w618]
              tunnel: w607 -> [w615 w622]
              tunnel: [w616 w621] -> w605
              tunnel: [w615 w620] -> w602
              tunnel: w606 -> [w614 w619]
              tunnel: [w614 w617] -> w599
              frame False {
              }
              frame True {
                n165 = for {
                  tunnel: w619 -> [w626] mode=indexing
                  tunnel: w618 -> [w625]
                  tunnel: [w624] -> w617 mode=indexing
                  n166 = for {
                    tunnel: w626 -> [w628]
                    tunnel: w625 -> [w629] mode=indexing
                    tunnel: [w627] -> w624 mode=indexing
                    n167 = Index Array(array=w628, index=w629) -> (element=w627:string)
                  }
                }
                n168 = for {
                  tunnel: w623 -> [w634]
                  tunnel: w618 -> [w630] mode=indexing
                  tunnel: w622 -> [w633]
                  tunnel: [w632] -> w621 mode=indexing
                  tunnel: [w631] -> w620 mode=indexing
                  n169 = Index Array(array=w633, index=w630) -> (element=w631:string)
                  n170 = Index Array(array=w634, index=w630) -> (element=w632:string)
                }
              }
            }
            n171 = for {
              tunnel: w599 -> [w613] mode=indexing
              tunnel: w598 -> [w612]
              tunnel: [w611] -> w597 mode=indexing
              n172 = Build Array (concatenate)(w613, w612) -> (w611:string[])
            }
            "Values" <- w597
            n173 = Build Array (concatenate)(w605, w604) -> (→"Column headers":string[])
            n174 = Build Array (concatenate)(w602, w601) -> (→"Header Comments":string[])
          }
          frame #9 {
          }
        }
      }
      frame "Add Adam Chs to header" {
        w641 = FALSE  # Email On Error?
        n175 = call "Channel_name_checker.vi"("Email On Error?"=w641, "Channel names"=w643) -> ("Channel names Out"=w642:string[])  [unwired: 1 out]
        n176 = for {
          tunnel: w642 -> [w665] mode=indexing
          tunnel: [w664] -> w658 mode=indexing
          tunnel: [w663] -> w657 mode=indexing
          tunnel: [w662] -> w656 mode=indexing
          n177 = call "Split_Ch_name.vi"("Ch name"=w665) -> ("Top level"=w664:string, "Middle"=w663:string, "Low level"=w662:string)
        }
        n178 = Array To Spreadsheet String(array=w646, 3:"%s" ("format string")) -> (spreadsheet string=w644:string)  [unwired: 1 out]
        n179 = Build Array(w658, w657, w656, w655, w654) -> (w652:string[][])
        n180 = Array To Spreadsheet String(array=w652, 3:"%s" ("format string")) -> (spreadsheet string=w645:string)  [unwired: 1 out]
        n181 = Concatenate Strings(w645, w644, "***************************************" ("Substring"), "\r\n", w648) -> (w651:string)
      }
      frame "Add Raw Data header info" {
        n182 = String Length(string=w670) -> (length=w672:i32)
        n183 = call "Raw_Data_File_Start_text.vi"("Header length"=w672) -> ("Start String"=w671:string)
        n184 = Concatenate Strings(w671, w670) -> (w669:string)
      }
      frame "Add Raw Data fr Tempory file" {
        w683 = 0  # Start to copy file at:
        n185 = global read "Constants_global.vi" "Data Folder Local"() -> (w687:path)
        n186 = Build Path(base path=w687, name or relative path="Tempory_Raw_Data_File.xls") -> (appended path=w684:path)
        n187 = call "Piece_file_Copy.vi"("File Start String"=w689, "Start to copy file at:"=w683, "Source File"=w684, "Target File"=w685) -> ()  [unwired: 1 out]
      }
    }
  }
  "Error String" <- w4
